vi "Generate Event.vi"(8 "Error In":errorcluster, 9 "Event Data":refnum<class "Event Data.lvclass">, 10 "Event Name":string, 11 "Event Source In":refnum<class "Event Source Actor.lvclass">) -> (0 "Error Out":errorcluster, 3 "Event Source Out":refnum<class "Event Source Actor.lvclass">)   [LabVIEW 2020, in "Event Source.lvlib" / "Event Source Actor.lvclass"]
doc: "This method generates/fires the Event wired to the input. Firing an event looks up all actors who Registered to listen to this Event and sends to them this Event on a Zero Coupling based message defined during Registration. Errors on broadcasting the event i.e. enqueuer of the registrant not existing, are ignored.\n\n<b>IMPORTANT</b> - Only call this method within actor core of your Event Source Actor. From helper loops call the Send Generate Event message to self. This is to make sure your actor works with all registered listeners."
uses:
  Event Source Actor.lvclass
  Event Data/Event Data.lvclass
  Event Source Actor.lvclass/Event Source Actor.ctl
  Template Receiver/Event Receiver Messages/Receive Event Msg/Receive Event Msg.lvclass/Receive Event Msg.ctl
  <vilib>/ActorFramework/Message Enqueuer/Message Enqueuer.lvclass/Message Enqueuer.ctl
  <vilib>/ActorFramework/Message Enqueuer/Enqueue.vi
  Template Receiver/Event Receiver Messages/Receive Event Msg/Receive Event Msg.lvclass
  C:/Program Files/National Instruments/LabVIEW 2020/vi.lib/ActorFramework/Message/Message.lvclass
  Program Files/National Instruments/LabVIEW 2020/resource/AFDebug/Generate Trace for Message.vi
  <vilib>/ActorFramework/Message Priority Queue/Priority Enqueue.vi
  Program Files/National Instruments/LabVIEW 2020/resource/AFDebug/AF Debug.lvlib
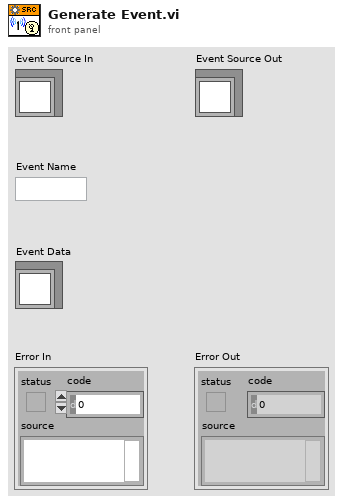
[diagram p1: front panel]
types:
  T1 = map{string, set{refnum<class "Message Enqueuer.lvclass">}}
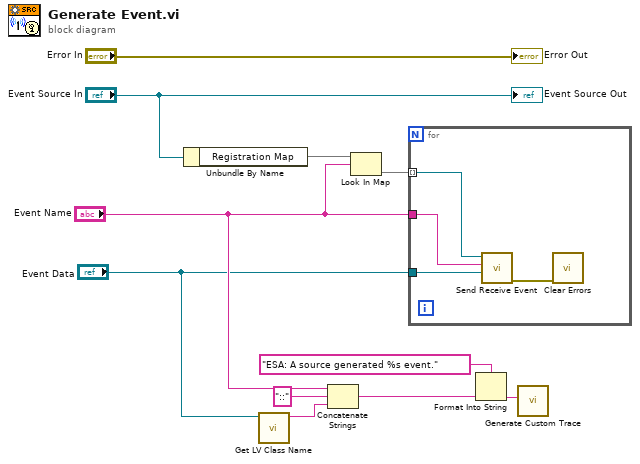
[diagram p0: block diagram]
diagram:
  n1 = Unbundle By Name("Event Source In") -> ("Registration Map"=w10:T1)
  n2 = call <vilib>:"Get LV Class Name.vi"("object"="Event Data") -> ("class name"=w4:string)  [unwired: 9 in, 1 out]
  n3 = Concatenate Strings("Event Name", "::" ("string"), w4) -> (w3:string)
  n4 = Look In Map(map=w10, key="Event Name") -> (value=w9:set{refnum<class "Message Enqueuer.lvclass">})  [unwired: 1 in, 1 out]
  n5 = for {
    tunnel: w9 -> [w14] mode=indexing
    tunnel: "Event Data" -> [w15]
    tunnel: "Event Name" -> [w13]
    n6 = call "Send Receive Event.vi"("Event Data"=w15, "Event Name"=w13, "Message Enqueuer"=w14) -> ("error out"=w12:errorcluster)  [unwired: 7 in, 1 out]
    n7 = call <vilib>:"Clear Errors.vi"("error in (no error)"=w12) -> ()  [unwired: 5 in, 2 out]
  }
  n8 = Format Into String(format string="ESA: A source generated %s event." ("Custom Action"), w3) -> (resulting string=w6:string)  [unwired: 2 in, 1 out]
  n9 = call "Generate Custom Trace.vi"("Custom Action"=w6) -> ()  [unwired: 11 in]
  "Error Out" <- "Error In"
  "Event Source Out" <- "Event Source In"
